vi "Create DAs.vi"(0 "reference in":refnum<class "Stand.lvclass">, 11 "error in (no error)":errorcluster) -> (4 "reference out":refnum<class "Stand.lvclass">, 15 "error out":errorcluster)   [LabVIEW 2019, in "Stand.lvclass"]
uses:
  Stand.lvclass
  C:/Users/ANENKOV_V1/Desktop/src/Proccess_class/Proccess.lvclass
  Stand.lvclass/Stand.ctl
  Proccess_class/Proccess.lvclass/Proccess.ctl
  Proccess_class/TAGs.ctl
  TypeDef/bool_setting.ctl
  DA_class/DA.lvclass
  Proccess_class/Proccess.lvclass
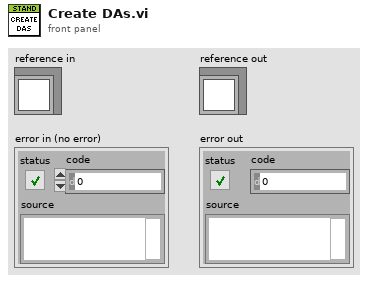
[diagram p1: front panel]
types:
  T1 = typedef "bool_setting.ctl" = cluster{"TON_ms":u32, "TOFF_ms":u32}
  T2 = typedef "Proccess.lvclass/TAGs.ctl" = cluster{"TAG":string, "PTAG":string, "DESC":string}
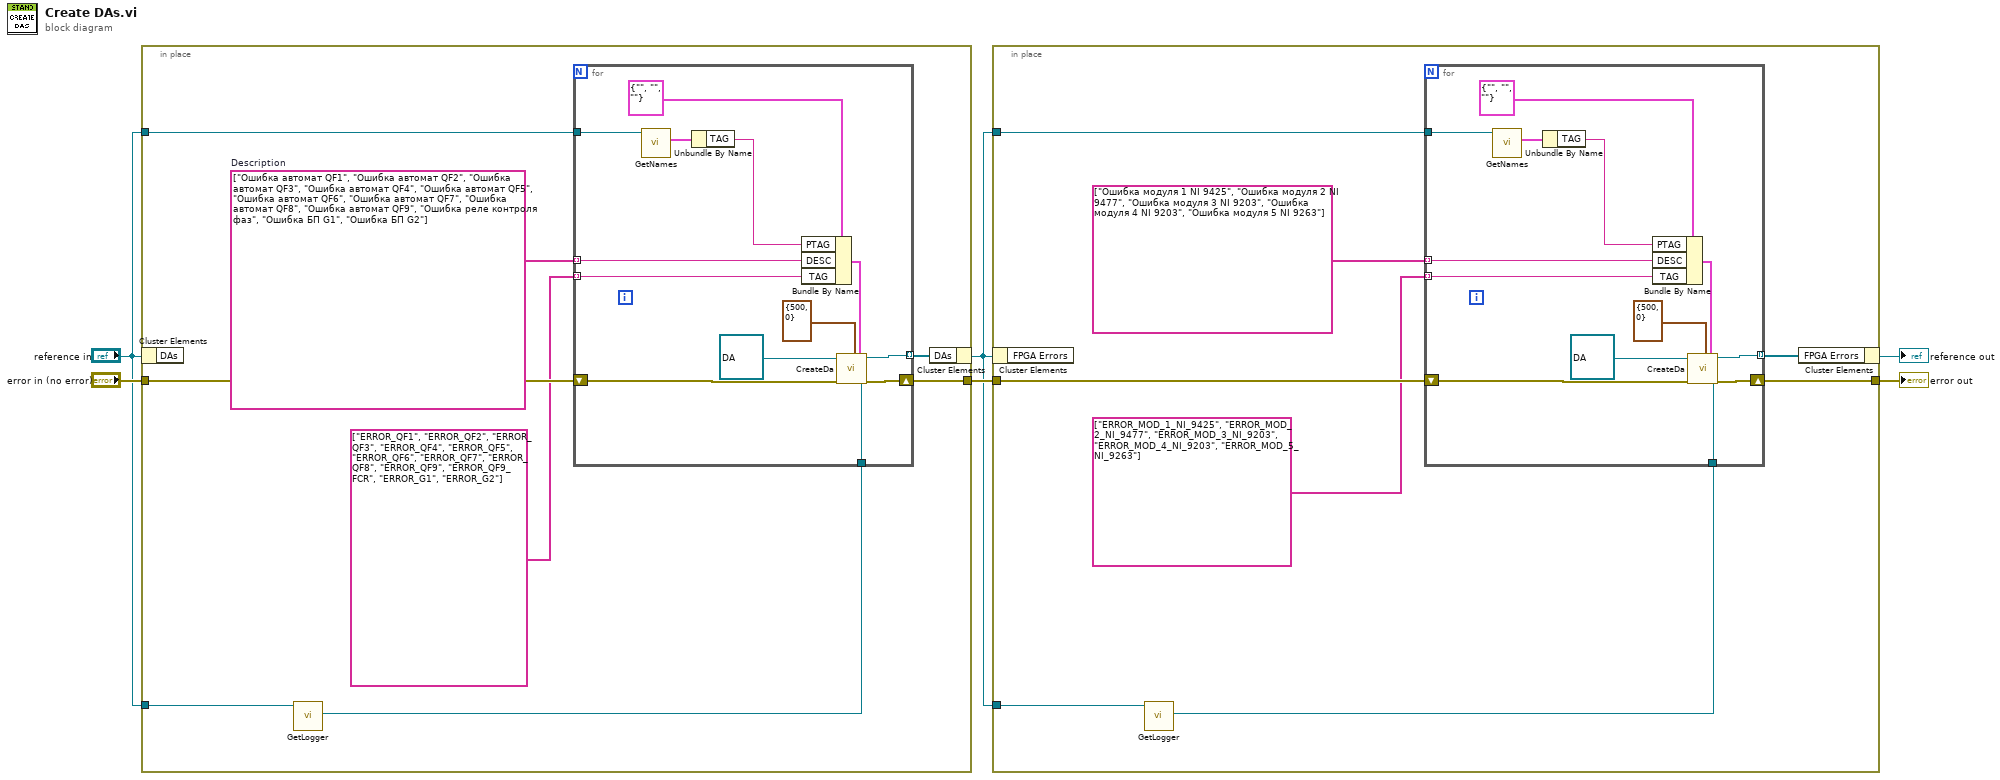
[diagram p0: block diagram]
diagram:
  n1 = in-place {
    in-place-border: "error in (no error)" -> [w14]
    in-place-border: "reference in" -> [w12]
    in-place-border: "reference in" -> [w11]
    in-place-border: [w8] -> w4
    w9 = string[] ["Ошибка автомат QF1", "Ошибка автомат QF2", "Ошибка автомат QF3", "Ошибка автомат QF4", "Ошибка автомат QF5", "Ошибка автомат QF6", "Ошибка автомат QF7", "Ошибка автомат QF8", "Ошибка автомат QF9", "Ошибка реле контроля фаз", "Ошибка БП G1", "Ошибка БП G2"]  # Description
    n2 = in-place-cluster #1("reference in") -> ()  [unwired: 1 out]
    n3 = call "GetLogger.vi"("Proccess in"=w11) -> ("Logger"=w10:refnum<class "Logger.lvclass">)  [unwired: 10 in]
    n4 = for {
      tunnel: [w26] -> w13 mode=indexing
      shift-right: [w25] -> w8
      shift-left: w14 -> [w27]
      tunnel: w9 -> [w22] mode=indexing
      tunnel: w12 -> [w19]
      tunnel: w10 -> [w18]
      tunnel: string[] ["ERROR_QF1", "ERROR_QF2", "ERROR_QF3", "ERROR_QF4", "ERROR_QF5", "ERROR_QF6", "ERROR_QF7", "ERROR_QF8", "ERROR_QF9", "ERROR_QF9_FCR", "ERROR_G1", "ERROR_G2"] -> [w15] mode=indexing
      n5 = call "GetNames.vi"("Proccess in"=w19) -> ("Tags"=w21:T2)  [unwired: 10 in]
      n6 = Unbundle By Name(w21) -> ("TAG"=w20:string)
      n7 = Bundle By Name(cluster=T2 {"TAG"="", "PTAG"="", "DESC"=""} ("Tags"), "PTAG"=w20, "DESC"=w22, "TAG"=w15) -> (w23:T2)
      n8 = call "CreateDa.vi"("Sig_DA in"=refnum<class "DA.lvclass"> refnum, "error in (no error)"=w27, "bool_setting"=T1 {"TON_ms"=500, "TOFF_ms"=0}, "Tags"=w23, "Logger"=w18) -> ("Sig_DA out"=w26:refnum<class "DA.lvclass">, "error out"=w25:errorcluster)  [unwired: 13 in]
    }
    n9 = in-place-cluster #1("DAs"=w13) -> (w1:refnum<class "Stand.lvclass">)
  }
  n10 = in-place {
    in-place-border: w4 -> [w35]
    in-place-border: w1 -> [w33]
    in-place-border: w1 -> [w32]
    in-place-border: [w30] -> w3
    n11 = in-place-cluster #2(w1) -> ()  [unwired: 1 out]
    n12 = call "GetLogger.vi"("Proccess in"=w32) -> ("Logger"=w31:refnum<class "Logger.lvclass">)  [unwired: 10 in]
    n13 = for {
      tunnel: [w47] -> w34 mode=indexing
      shift-right: [w46] -> w30
      shift-left: w35 -> [w48]
      tunnel: string[] ["Ошибка модуля 1 NI 9425", "Ошибка модуля 2 NI 9477", "Ошибка модуля 3 NI 9203", "Ошибка модуля 4 NI 9203", "Ошибка модуля 5 NI 9263"] -> [w43] mode=indexing
      tunnel: w33 -> [w40]
      tunnel: w31 -> [w39]
      tunnel: string[] ["ERROR_MOD_1_NI_9425", "ERROR_MOD_2_NI_9477", "ERROR_MOD_3_NI_9203", "ERROR_MOD_4_NI_9203", "ERROR_MOD_5_NI_9263"] -> [w36] mode=indexing
      n14 = call "GetNames.vi"("Proccess in"=w40) -> ("Tags"=w42:T2)  [unwired: 10 in]
      n15 = Unbundle By Name(w42) -> ("TAG"=w41:string)
      n16 = Bundle By Name(cluster=T2 {"TAG"="", "PTAG"="", "DESC"=""} ("Tags"), "PTAG"=w41, "DESC"=w43, "TAG"=w36) -> (w44:T2)
      n17 = call "CreateDa.vi"("Sig_DA in"=refnum<class "DA.lvclass"> refnum, "error in (no error)"=w48, "bool_setting"=T1 {"TON_ms"=500, "TOFF_ms"=0}, "Tags"=w44, "Logger"=w39) -> ("Sig_DA out"=w47:refnum<class "DA.lvclass">, "error out"=w46:errorcluster)  [unwired: 13 in]
    }
    n18 = in-place-cluster #2("FPGA Errors"=w34) -> (→"reference out":refnum<class "Stand.lvclass">)
  }
  "error out" <- w3
